vi "initializeDisplay.vi"(8 "error in (no error)":errorcluster, 10 "stringControlRefnum":refnum<vi>, 11 "TextDisplay Class in":refnum<class "TextDisplay Class.lvclass">) -> (0 "error out":errorcluster, 3 "TextDisplay Class out":refnum<class "TextDisplay Class.lvclass">)   [LabVIEW 2019, in "TextDisplay Class.lvclass"]
uses:
  TextDisplay Class.lvclass
  TextDisplay Class.lvclass/TextDisplay Class.ctl
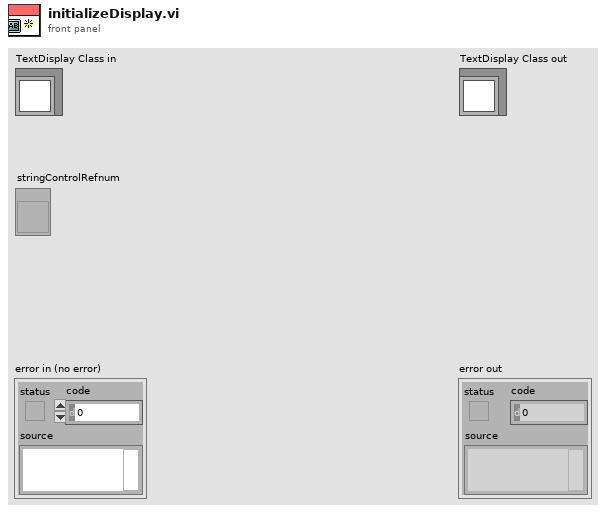
[diagram p1: front panel]
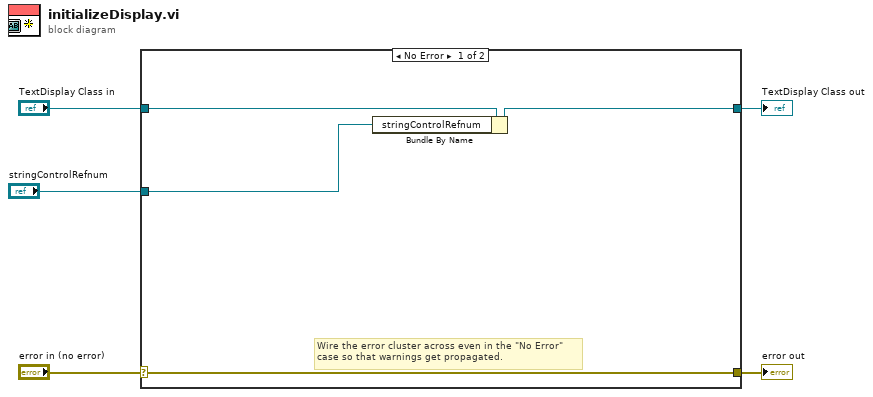
[diagram p0: block diagram]
diagram:
  n1 = case shown="No Error" "error in (no error)" {
    selector: "error in (no error)" -> [w8 w11]
    tunnel: [w8 w11] -> w4
    tunnel: [w7 w10] -> w2
    tunnel: "TextDisplay Class in" -> [w9 w10]
    tunnel: "stringControlRefnum" -> [w6 _]
    frame No Error {
      # "Wire the error cluster across even in the \"No Error\"\ncase so that warnings get propagated."
      n2 = Bundle By Name(cluster=w9, "stringControlRefnum"=w6) -> (w7:refnum<class "TextDisplay Class.lvclass">)
    }
    frame Error {
    }
  }
  "error out" <- w4
  "TextDisplay Class out" <- w2
